vi "Encapsulate in a bat.vi"(7 "Overwrite?":bool=TRUE, 8 "error in (no error)":errorcluster, 10 "command":string, 11 "Kasli Wrapper in":refnum<class "Kasli Wrapper 2.0.lvclass">) -> (0 "error out":errorcluster, 2 "bat out":string, 3 "Kasli Wrapper out":refnum<class "Kasli Wrapper 2.0.lvclass">)   [LabVIEW 2020, in "Kasli Wrapper 2.0.lvlib" / "Kasli Wrapper 2.0.lvclass"]
doc: "Submit script to the Master for execution. If Dummy flag is set to true, the script is submitted with artiq_run command and the DAQ flag is ignored (running without connection to the DAQ). Otherwise, if the DAQ flag is set to true, the script will start DAQ connection. \nOverwrite flag is used for selecting the .bat file name for storring the submit command. If it is true, then the Batman.bat and Robin.bat are used for submitting scripts to standard and dummy Kaslis respectively. Otherwise, a .bat file is created with an unique GUID as the name."
uses:
  Kasli Wrapper 2.0.lvclass
  Kasli Wrapper 2.0.lvclass/Kasli Wrapper 2.0.ctl
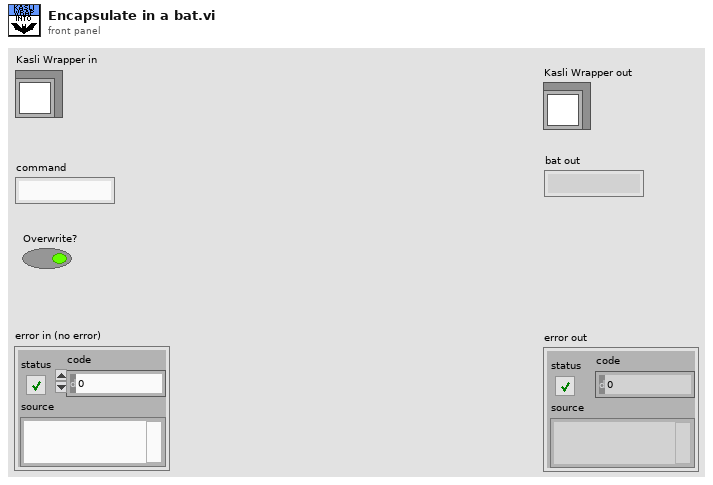
[diagram p1: front panel]
types:
  T1 = enum16{"open", "replace", "create", "open or create", "replace or create", "replace or create with confirmation"}
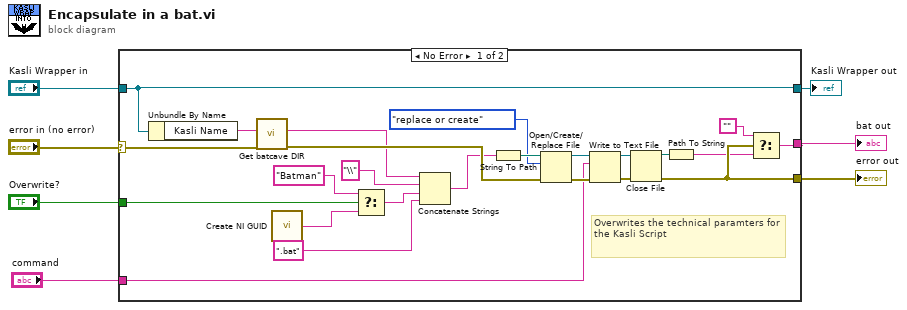
[diagram p0: block diagram]
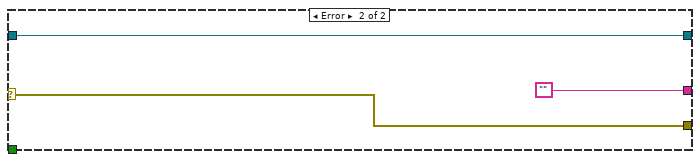
[diagram p2: hidden frame]
diagram:
  n1 = case shown="No Error" "error in (no error)" {
    selector: "error in (no error)" -> [w13 w34]
    tunnel: [w31 w34] -> w6
    tunnel: [w15 ""] -> w5
    tunnel: "Overwrite?" -> [w18 _]
    tunnel: "Kasli Wrapper in" -> [w9 w32]
    tunnel: [w9 w32] -> w2
    tunnel: "command" -> [w8 _]
    frame No Error {
      # "Overwrites the technical paramters for the Kasli Script"
      n2 = Unbundle By Name(w9) -> ("Kasli Name"=w11:string)
      n3 = call "Get batcave DIR.vi"("error in (no error)"=w13, "relative path"=w11) -> ("error out"=w30:errorcluster, "Batcave DIR"=w10:string)  [unwired: 4 in]
      n4 = call <vilib>:"Create NI GUID.vi"() -> ("NI GUID"=w16:string)
      n5 = Select(t="Batman" ("f"), s=w18, f=w16) -> (s? t:f=w17:string)
      n6 = Concatenate Strings(w10, "\\" ("string"), w17, ".bat" ("string")) -> (w27:string)
      n7 = String To Path(string=w27) -> (path=w29:path)
      n8 = Open/Create/Replace File(file path (use dialog)=w29, error in=w30, operation (0:open)=T1."replace or create") -> (refnum out=w25:refnum<file>, error out=w24:errorcluster)  [unwired: 3 in, 1 out]
      n9 = Write to Text File(file (use dialog)=w25, text=w8, error in=w24) -> (refnum out=w23:refnum<file>, error out=w22:errorcluster)  [unwired: 1 in, 1 out]
      n10 = Close File(refnum=w23, error in=w22) -> (path=w21:path, error out=w31:errorcluster)
      n11 = Path To String(path=w21) -> (string=w20:string)
      n12 = Select(t="", s=w31, f=w20) -> (s? t:f=w15:string)
    }
    frame Error {
    }
  }
  "error out" <- w6
  "bat out" <- w5
  "Kasli Wrapper out" <- w2
